vi "Read Region Position Fixture ID.vi"(8 "error in (no error)":errorcluster, 11 "Fixture in":refnum<class "Fixture.lvclass">) -> (0 "error out":errorcluster, 2 "Cluster":T1, 3 "Fixture out":refnum<class "Fixture.lvclass">)   [LabVIEW 2021, in "Fixture.lvclass"]
uses:
  Fixture.lvclass
  Fixture.lvclass/Fixture.ctl
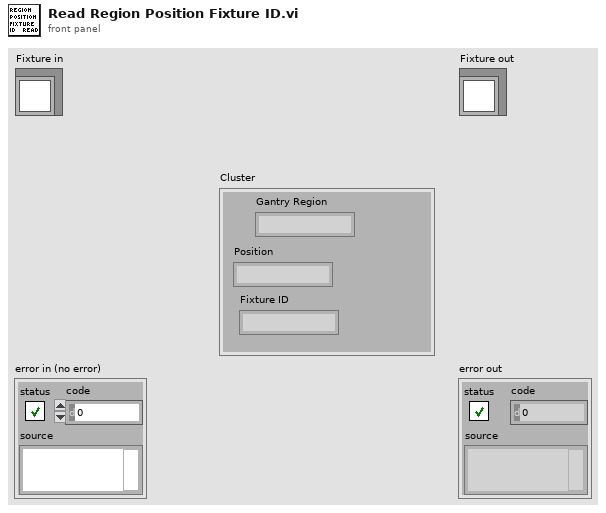
[diagram p1: front panel]
types:
  T1 = cluster{"Gantry Region":string, "Position":string, "Fixture ID":string}
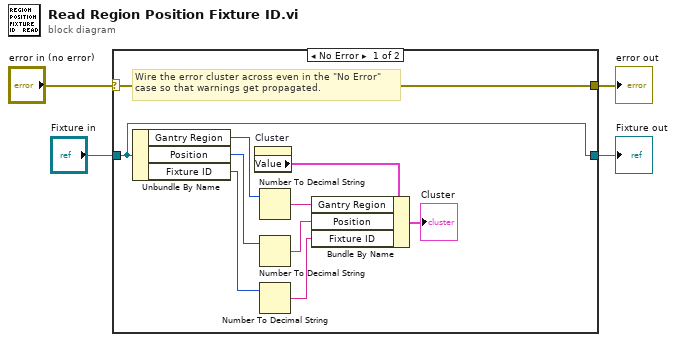
[diagram p0: block diagram]
diagram:
  n1 = case shown="No Error" "error in (no error)" {
    selector: "error in (no error)" -> [w14 w16]
    tunnel: [w14 w16] -> w3
    tunnel: [w13 w15] -> w1
    tunnel: "Fixture in" -> [w13 w15]
    frame No Error {
      # "Wire the error cluster across even in the \"No Error\"\ncase so that warnings get propagated."
      n2 = Unbundle By Name(w13) -> ("Gantry Region"=w12:i32, "Position"=w11:i32, "Fixture ID"=w10:i32)
      n3 = property on="Cluster" class="Clust (strict)"() -> ("Value"=w9:T1)  [unwired: 2 in, 2 out]
      n4 = Number To Decimal String(number=w12) -> (decimal integer string=w7:string)  [unwired: 1 in]
      n5 = Number To Decimal String(number=w11) -> (decimal integer string=w6:string)  [unwired: 1 in]
      n6 = Number To Decimal String(number=w10) -> (decimal integer string=w5:string)  [unwired: 1 in]
      n7 = Bundle By Name(cluster=w9, "Gantry Region"=w7, "Position"=w6, "Fixture ID"=w5) -> (→"Cluster":T1)
    }
    frame Error {
    }
  }
  "error out" <- w3
  "Fixture out" <- w1
